vi "DisconnectCore.vi"(8 "error in (no error)":errorcluster, 11 "GRPCClient in":refnum<class "MicronGRPCClient.lvclass">) -> (0 "error out":errorcluster, 3 "GRPCClient out":refnum<class "MicronGRPCClient.lvclass">)   [LabVIEW 2019, in "MicronGRPCClient.lvclass"]
uses:
  MicronGRPCClient.lvclass
  MicronGRPCClient.lvclass/MicronGRPCClient.ctl
  Generated/MicronGRPCGeneratedClient/MicronGRPCGeneratedClient.lvlib
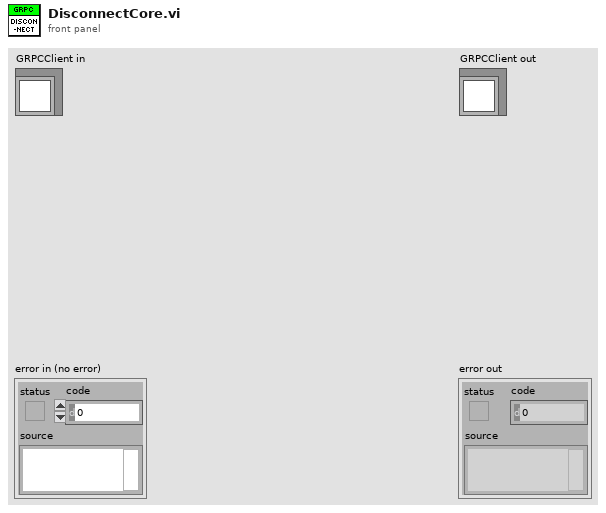
[diagram p1: front panel]
types:
  T1 = typedef "grpc-lvsupport-release.lvlib/grpcId.ctl" = u64
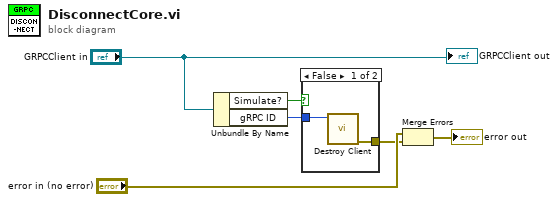
[diagram p0: block diagram]
diagram:
  n1 = Unbundle By Name("GRPCClient in") -> ("Simulate?"=w4:bool, "gRPC ID"=w5:T1)
  n2 = case shown="False" w4 {
    tunnel: [w8 _] -> w1
    tunnel: w5 -> [w7 _]
    frame False {
      n3 = call "Destroy Client.vi"("gRPC ID"=w7) -> ("error out"=w8:errorcluster)  [unwired: 10 in]
    }
    frame True {
    }
  }
  n4 = Merge Errors("error in (no error)", w1) -> (→"error out":errorcluster)
  "GRPCClient out" <- "GRPCClient in"
